vi "Update Instrument Status.vi"(8 "error in (no error)":errorcluster, 9 "Value (0)":u32, 10 "Instrument Status (0: Standard Event Status Enable Register)":u32(ring) items=["Standard Event Status Enable Register", "Service Request Enable Register"], 11 "VISA resource name":refnum<visa-resource-name>) -> (0 "error out":errorcluster, 3 "VISA resource name out":refnum<visa-resource-name>)   [LabVIEW 2022 SP3, in "MagnaDC.lvlib"]
uses:
  MagnaDC.lvlib
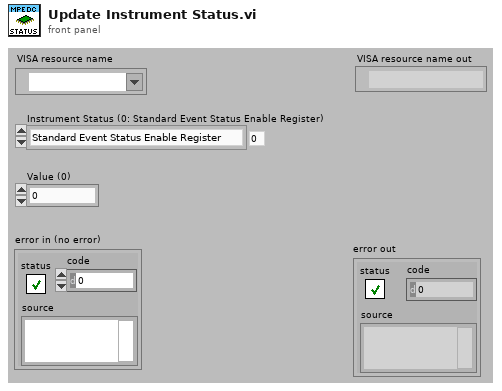
[diagram p1: front panel]
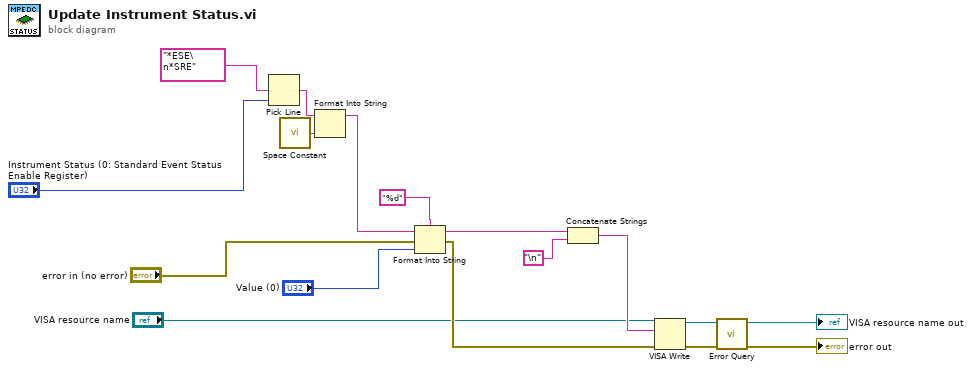
[diagram p0: block diagram]
diagram:
  n1 = Pick Line(multi-line string="*ESE\n*SRE", line index="Instrument Status (0: Standard Event Status Enable Register)") -> (output string=w3:string)  [unwired: 1 in]
  n2 = call <vilib>:"Space Constant.vi"() -> ("String"=w4:string)
  n3 = Format Into String(initial string=w3, w4) -> (resulting string=w2:string)  [unwired: 2 in, 1 out]
  n4 = Format Into String(format string="%d", initial string=w2, error in="error in (no error)", "Value (0)") -> (resulting string=w10:string, error out=w9:errorcluster)
  n5 = Concatenate Strings(w10, "\n") -> (w12:string)
  n6 = VISA Write(VISA resource name="VISA resource name", write buffer=w12, error in (no error)=w9) -> (VISA resource name out=w15:refnum<visa-resource-name>, error out=w14:errorcluster)  [unwired: 1 out]
  n7 = call "Error Query.vi"("error in (no error)"=w14, "VISA resource name"=w15) -> ("error out"=→"error out":errorcluster, "VISA resource name out"=→"VISA resource name out":refnum<visa-resource-name>)  [unwired: 6 in, 2 out]
